vi "random subvi.vi"() -> ()   [LabVIEW 2014]
panel:
  out "Numeric":dbl
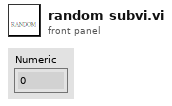
[diagram p1: front panel]
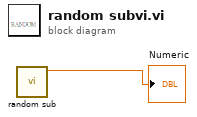
[diagram p0: block diagram]
diagram:
  n1 = call "random sub.vi"() -> ("Numeric"=→"Numeric":dbl)  [unwired: 11 in]
